vi "Teleop.vi"(10 "Match Info":T1={"Autonomous Elapsed Seconds"=0.0, "TeleOp Elapsed Seconds"=0.0, "Disabled Elapsed Seconds"=0.0, "Visited Autonomous"=FALSE, "Visited TeleOp"=FALSE, "Visited Disabled"=FALSE, "Autonomous Settings"={"Autonomous Style"=enum."Independent", "VI Refnum"=refnum}}, 11 "Call Context":T2) -> ()   [LabVIEW 2016]
doc: "This VI is called for each enabled TeleOp packet received from the DS. It is typically used to read from joysticks and other inputs and update I/O or setpoints for timed control loops. It should complete and return within 20 milliseconds or risk missing DS packets."
uses:
  <vilib>/Rock Robotics/WPI/DriverStation/WPI_DriverStationDerivedRobotMode.ctl
  <vilib>/Rock Robotics/WPI/DriverStation/WPI_DriverStationMatch Info.ctl
  <vilib>/Rock Robotics/WPI/ThirdParty/CanMotor/TalonSRX/WPI_CANTalonSRX_APIControlMode.ctl
  <vilib>/Rock Robotics/WPI/Utilities/WPI_GetSetVariantRefNum.vi
  <vilib>/Rock Robotics/Network Tables/NT Write Boolean Array.vi
  <vilib>/Rock Robotics/Network Tables/NT Write Numeric Array.vi
  <vilib>/Rock Robotics/Network Tables/NT Write String Array.vi
  <vilib>/Rock Robotics/Network Tables/NT Write Number.vi
  <vilib>/Rock Robotics/Network Tables/NT Read Number.vi
  Framework/Robot Global Data.vi
  <vilib>/Rock Robotics/Network Tables/NT Write Boolean.vi
panel:
  out "Percent Vbus?":bool
  out "Right Bumper Latched Driver":bool
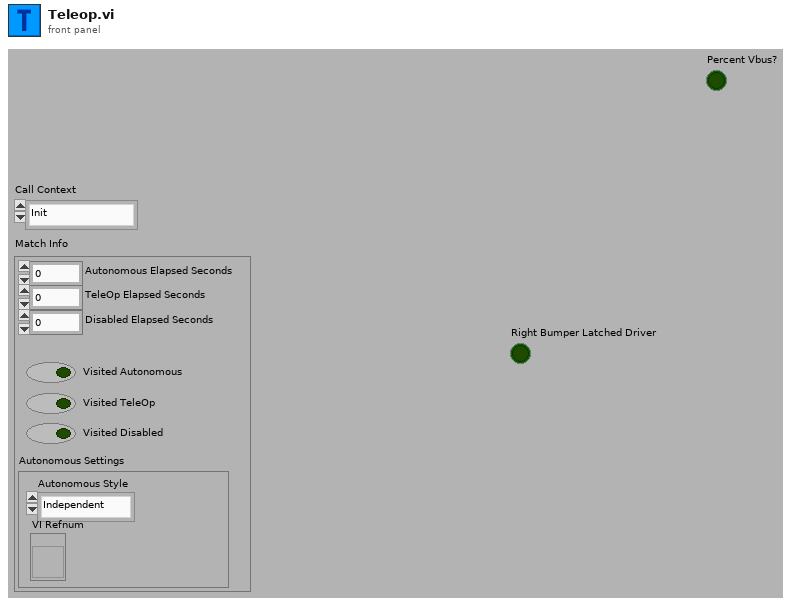
[diagram p1: front panel]
types:
  T1 = typedef "WPI_DriverStationMatch Info.ctl" = cluster{"Autonomous Elapsed Seconds":dbl, "TeleOp Elapsed Seconds":dbl, "Disabled Elapsed Seconds":dbl, "Visited Autonomous":bool, "Visited TeleOp":bool, "Visited Disabled":bool, "Autonomous Settings":cluster{"Autonomous Style":enum16{"Iterative", "Independent"}, "VI Refnum":refnum<vi>}}
  T2 = typedef "WPI_DriverStationDerivedRobotMode.ctl" = enum16{"Init", "Execute", "Stop"}
  T3 = typedef "WPI_JoystickDevRef.ctl" = cluster{"Device":T4}
  T4 = typedef "WPI_JoystickDeviceEnum.ctl" = enum16{"USB 0", "USB 1", "USB 2", "USB 3", "USB 4", "USB 5"}
  T5 = typedef "WPI_MotorControlDeviceRef.ctl" = cluster{"DeviceStatus":errorcluster, "Type":T6, "PWM":cluster{"PWM Channel":T7, "DeadBand":T8}, "CAN":cluster{"Device Number":u8, "SetOutput VI Ref":variant, "GetOutput VI Ref":variant, "Enable VI Ref":variant, "Disable VI Ref":variant, "Data":variant}, "Invert":bool}
  T6 = typedef "WPI_MotorControlType.ctl" = enum16{"PWM", "CAN"}
  T7 = typedef "FPGA_DIOPWMChannel.ctl" = enum8{"PWM 0", "PWM 1", "PWM 2", "PWM 3", "PWM 4", "PWM 5", "PWM 6", "PWM 7", "PWM 8", "PWM 9", "PWM MXP 0", "PWM MXP 1", "PWM MXP 2", "PWM MXP 3", "PWM MXP 4", "PWM MXP 5", "PWM MXP 6", "PWM MXP 7", "PWM MXP 8", "PWM MXP 9", "Invalid"}
  T8 = typedef "WPI_PWMDeadband.ctl" = cluster{"Name":string, "maxPositivePwm":i32, "minPositivePwm":i32, "centerPwm":i32, "maxNegativePwm":i32, "minNegativePwm":i32, "angularRange":u16}
  T9 = typedef "WPI_DigitalInputDevRef.ctl" = cluster{"DevStatus":errorcluster, "DIO Channel":T10}
  T10 = typedef "FPGA_DIOChannel.ctl" = enum8{"DIO 0", "DIO 1", "DIO 2", "DIO 3", "DIO 4", "DIO 5", "DIO 6", "DIO 7", "DIO 8", "DIO 9", "DIO MXP 0", "DIO MXP 1", "DIO MXP 2", "DIO MXP 3", "DIO MXP 4", "DIO MXP 5", "DIO MXP 6", "DIO MXP 7", "DIO MXP 8", "DIO MXP 9", "DIO MXP 10", "DIO MXP 11", "DIO MXP 12", "DIO MXP 13", "DIO MXP 14", "DIO MXP 15", "SPI Port CS1", "SPI Port CS2", "SPI Port CS3", "SPI Port MISO", "SPI Port MOSI", "Invalid"}
  T11 = typedef "WPI_RobotDriveDevRef.ctl" = cluster{"DevStatus":errorcluster, "Motors[]":T5[], "Square Inputs":bool, "Max Output":dbl}
  T12 = typedef "WPI_CANTalonSRX_APIControlMode.ctl" = enum8{"Percent VBus", "Speed", "Position", "Slave", "Unchanged / Invalid", "Voltage Compensation", "Current", "Motion Profile", "Motion Magic"}
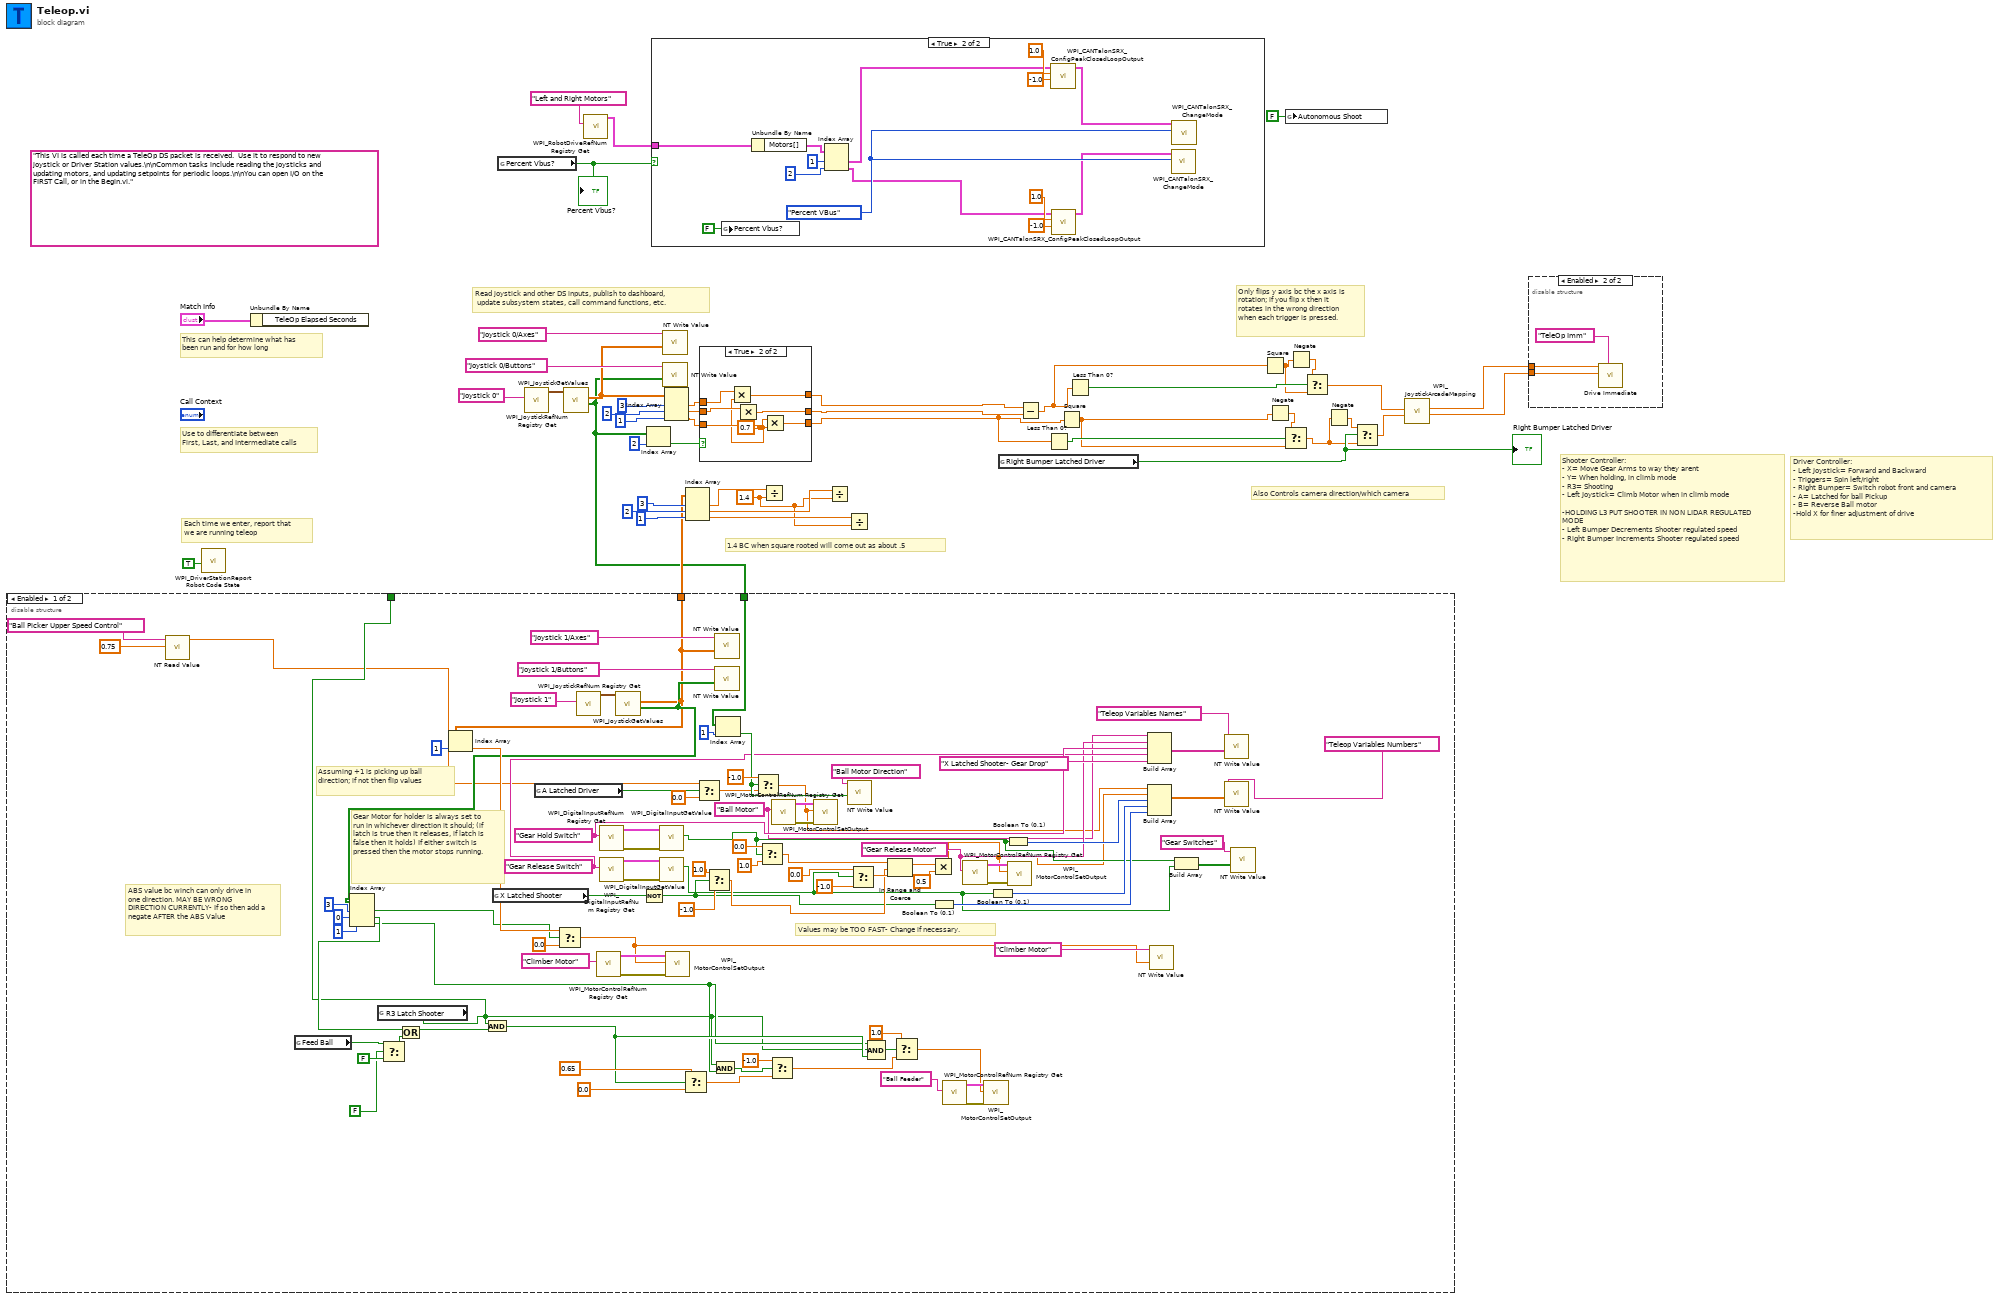
[diagram p0: block diagram]
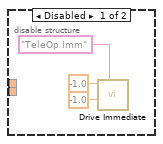
[diagram p4: hidden frame]
diagram:
  w13 = 1.4 ("y")
  (unwired) "This VI is called each time a TeleOp DS packet is received.  Use it to respond to new joystick or Driver Station values.\n\nCommon tasks include reading the joysticks and updating motors, and updating setpoints for periodic loops.\n\nYou can open I/O on the FIRST Call, or in the Begin.vi."
  # "1.4 BC when square rooted will come out as about .5"
  # "Driver Controller:\n- Left Joystick= Forward and Backward\n- Triggers= Spin left/right\n- Right Bumper= Switch robot front and camera\n- A= Latched for ball Pickup\n- B= Reverse Ball motor\n-Hold X for finer adjustment of drive"
  # "Shooter Controller:\n- X= Move Gear Arms to way they arent\n- Y= When holding, in climb mode\n- R3= Shooting\n- Left Joystick= Climb Motor when in climb mode\n\n-HOLDING L3 PUT SHOOTER IN NON LIDAR REGULATED MODE\n- Left Bumper Decrements Shooter regulated speed\n- Right Bumper Increments Shooter regulated speed"
  # "Only flips y axis bc the x axis is rotation; if you flip x then it rotates in the wrong direction when each trigger is pressed."
  # "Also Controls camera direction/which camera"
  # "Read joystick and other DS inputs, publish to dashboard,\n update subsystem states, call command functions, etc."
  # "Each time we enter, report that\nwe are running teleop"
  # "Use to differentiate between\nFirst, Last, and Intermediate calls"
  # "This can help determine what has\nbeen run and for how long"
  n1 = call <vilib>:"WPI_DriverStationReport Robot Code State.vi"("TeleOp"=TRUE ("Autonomous")) -> ()  [unwired: 10 in, 1 out]
  n2 = Unbundle By Name("Match Info") -> ()  [unwired: 1 out]
  n3 = global read "Robot Global Data.vi" "Percent Vbus?"() -> (w2:bool)
  "Percent Vbus?" <- w2
  n4 = call <vilib>:"WPI_JoystickRefNum Registry Get.vi"("refnum name"="Joystick 0") -> ("JoystickDevRef"=w42:T3)  [unwired: 1 in, 9 out]
  n5 = call <vilib>:"WPI_JoystickGetValues.vi"("JoystickDevRef"=w42) -> ("Buttons"=w12:bool[], "Axes"=w40:dbl[])  [unwired: 6 in, 3 out]
  n6 = disable-structure shown="Enabled" {
    disable-tunnel: w12 -> [w80 _]
    disable-tunnel: [w50 _] -> _
    disable-tunnel: [w66 _] -> w17
    frame Enabled {
      w110 = "Gear Release Switch" ("refnum name")
      w112 = "Gear Hold Switch" ("refnum name")
      w74 = "Gear Release Motor" ("refnum name")
      w73 = "Ball Motor" ("refnum name")
      # "ABS value bc winch can only drive in one direction. MAY BE WRONG DIRECTION CURRENTLY- If so then add a negate AFTER the ABS Value"
      # "Gear Motor for holder is always set to run in whichever direction it should; (if latch is true then it releases, if latch is false then it holds) If either switch is pressed then the motor stops running."
      # "Values may be TOO FAST- Change if necessary."
      # "Assuming +1 is picking up ball direction; if not then flip values"
      n7 = call-poly <vilib>:"NT Read Value.vi"("Default Value"=0.75, "Name"="Ball Picker Upper Speed Control") -> ("Numeric"=w49:dbl)  [unwired: 8 in, 1 out]
      n8 = global read "Robot Global Data.vi" "Feed Ball"() -> (w69:bool)
      n9 = global read "Robot Global Data.vi" "R3 Latch Shooter"() -> (w50:bool)
      n10 = Select(t=w69, s=FALSE ("AutoFeed Balls"), f=FALSE) -> (s? t:f=w70:bool)
      n11 = global read "Robot Global Data.vi" "X Latched Shooter"() -> (w81:bool)
      n12 = global read "Robot Global Data.vi" "A Latched Driver"() -> (w83:bool)
      n13 = call <vilib>:"WPI_JoystickRefNum Registry Get.vi"("refnum name"="Joystick 1") -> ("JoystickDevRef"=w133:T3)  [unwired: 1 in, 9 out]
      n14 = call <vilib>:"WPI_MotorControlRefNum Registry Get.vi"("refnum name"="Climber Motor") -> ("error out"=w120:errorcluster, "MotorControlDevRef"=w78:T5)  [unwired: 9 in]
      n15 = call <vilib>:"WPI_DigitalInputRefNum Registry Get.vi"("refnum name"=w112) -> ("error out"=w124:errorcluster, "DigitalInputDevRef"=w123:T9)  [unwired: 9 in]
      n16 = call <vilib>:"WPI_DigitalInputRefNum Registry Get.vi"("refnum name"=w110) -> ("error out"=w122:errorcluster, "DigitalInputDevRef"=w121:T9)  [unwired: 9 in]
      n17 = call <vilib>:"WPI_JoystickGetValues.vi"("JoystickDevRef"=w133) -> ("Buttons"=w86:bool[], "Axes"=w66:dbl[])  [unwired: 6 in, 3 out]
      n18 = Index Array(array=w86, index #1=3 ("index"), index #2=0 ("index"), index #3=1 ("index")) -> (element #1=w85:bool, element #2=w75:bool, element #3=w51:bool)
      n19 = Or(x=w75, y=w70) -> (x .or. y?=w71:bool)
      n20 = Index Array(array=w66, index=1) -> (element=w88:dbl)
      n21 = And(x=w50, y=w71) -> (x .and. y?=w53:bool)
      n22 = Select(t=w88, s=w85, f=0.0) -> (s? t:f=w77:dbl)
      n23 = Not(x=w81) -> (.not. x?=w79:bool)
      n24 = call <vilib>:"WPI_DigitalInputGetValue.vi"("error in (no error)"=w124, "DigitalInputDevRef"=w123) -> ("Value"=w93:bool)  [unwired: 7 in, 2 out]
      n25 = call <vilib>:"WPI_DigitalInputGetValue.vi"("error in (no error)"=w122, "DigitalInputDevRef"=w121) -> ("Value"=w92:bool)  [unwired: 7 in, 2 out]
      n26 = call <vilib>:"WPI_MotorControlSetOutput.vi"("error in (no error)"=w120, "Output"=w77, "MotorControlDevRef"=w78) -> ()  [unwired: 6 in, 3 out]
      n27 = Select(t=0.65 ("Ball Feeder Speed"), s=w53, f=0.0) -> (s? t:f=w60:dbl)
      n28 = Select(t=w49, s=w83, f=0.0) -> (s? t:f=w84:dbl)
      n29 = Select(t=1.0, s=w79, f=-1.0) -> (s? t:f=w94:dbl)
      n30 = And(x=w50, y=w51) -> (x .and. y?=w52:bool)
      n31 = call-poly <vilib>:"NT Write Value.vi"("Numeric Array"=w66, "Name"="Joystick 1/Axes") -> ()  [unwired: 9 in, 1 out]
      n32 = call-poly <vilib>:"NT Write Value.vi"("Boolean Array"=w86, "Name"="Joystick 1/Buttons") -> ()  [unwired: 9 in, 1 out]
      n33 = Index Array(array=w80, index=1) -> (element=w118:bool)
      n34 = Select(t=-1.0 ("Backward"), s=w118, f=w84) -> (s? t:f=w46:dbl)
      n35 = Select(t=0.0, s=w93, f=1.0) -> (s? t:f=w95:dbl)
      n36 = Select(t=-1.0, s=w52, f=w60) -> (s? t:f=w55:dbl)
      n37 = call <vilib>:"WPI_MotorControlRefNum Registry Get.vi"("refnum name"=w73) -> ("error out"=w130:errorcluster, "MotorControlDevRef"=w129:T5)  [unwired: 9 in]
      n38 = call <vilib>:"WPI_MotorControlSetOutput.vi"("error in (no error)"=w130, "Output"=w46, "MotorControlDevRef"=w129) -> ()  [unwired: 6 in, 3 out]
      n39 = call-poly <vilib>:"NT Write Value.vi"("Boolean"=w118, "Name"="Ball Motor Direction") -> ()  [unwired: 9 in, 1 out]
      n40 = Select(t=0.0, s=w92, f=-1.0) -> (s? t:f=w100:dbl)
      n41 = Compound Arithmetic op=AND(w51, w50, w53) -> (w56:bool)
      n42 = In Range and Coerce(upper limit=w95, x=w94, lower limit=w100) -> (coerced(x)=w91:dbl)  [unwired: 1 out]
      n43 = Select(t=1.0, s=w56, f=w55) -> (s? t:f=w57:dbl)
      n44 = Multiply(x=w91, y=0.5) -> (x*y=w72:dbl)
      n45 = Boolean To (0,1)(Boolean=w79) -> (0, 1=w107:i16)
      n46 = call <vilib>:"WPI_MotorControlRefNum Registry Get.vi"("refnum name"="Ball Feeder") -> ("error out"=w65:errorcluster, "MotorControlDevRef"=w64:T5)  [unwired: 9 in]
      n47 = call <vilib>:"WPI_MotorControlRefNum Registry Get.vi"("refnum name"=w74) -> ("error out"=w126:errorcluster, "MotorControlDevRef"=w125:T5)  [unwired: 9 in]
      n48 = call <vilib>:"WPI_MotorControlSetOutput.vi"("error in (no error)"=w65, "Output"=w57, "MotorControlDevRef"=w64) -> ()  [unwired: 6 in, 3 out]
      n49 = Boolean To (0,1)(Boolean=w92) -> (0, 1=w109:i16)
      n50 = Boolean To (0,1)(Boolean=w93) -> (0, 1=w111:i16)
      n51 = call <vilib>:"WPI_MotorControlSetOutput.vi"("error in (no error)"=w126, "Output"=w72, "MotorControlDevRef"=w125) -> ()  [unwired: 6 in, 3 out]
      n52 = Build Array(w73, w74, w112, w110, "X Latched Shooter- Gear Drop") -> (w115:string[])
      n53 = Build Array(w46, w72, w111, w109, w107) -> (w114:dbl[])
      n54 = call-poly <vilib>:"NT Write Value.vi"("Numeric"=w77, "Name"="Climber Motor") -> ()  [unwired: 9 in, 1 out]
      n55 = Build Array(w93, w92) -> (w104:bool[])
      n56 = call-poly <vilib>:"NT Write Value.vi"("String Array"=w115, "Name"="Teleop Variables Names") -> ()  [unwired: 9 in, 1 out]
      n57 = call-poly <vilib>:"NT Write Value.vi"("Numeric Array"=w114, "Name"="Teleop Variables Numbers") -> ()  [unwired: 9 in, 1 out]
      n58 = call-poly <vilib>:"NT Write Value.vi"("Boolean Array"=w104, "Name"="Gear Switches") -> ()  [unwired: 9 in, 1 out]
    }
    frame Disabled {
    }
  }
  n59 = call <vilib>:"WPI_RobotDriveRefNum Registry Get.vi"("refnum name"="Left and Right Motors") -> ("RobotDriveDevRef"=w5:T11)  [unwired: 9 in, 1 out]
  n60 = Index Array(array=w12, index=2) -> (element=w7:bool)
  n61 = case shown="True" w2 {
    tunnel: w5 -> [_ w143]
    frame False {
    }
    frame True {
      w145 = WPI_CANTalonSRX_APIControlMode."Percent VBus" ("Control Mode")
      n62 = global write "Robot Global Data.vi" "Percent Vbus?"(FALSE ("Percent Vbus?")) -> ()
      n63 = Unbundle By Name(w143) -> ("Motors[]"=w148:T5[])
      n64 = Index Array(array=w148, index #1=1 ("index"), index #2=2 ("index")) -> (element #1=w137:T5, element #2=w136:T5)
      n65 = call <vilib>:"WPI_CANTalonSRX_ConfigPeakClosedLoopOutput.vi"("Reverse Peak Output"=-1.0, "Forward Peak Output"=1.0, "CAN Talon SRX Ref"=w137) -> ("CAN Talon SRX Ref"=w138:T5)  [unwired: 7 in, 1 out]
      n66 = call <vilib>:"WPI_CANTalonSRX_ConfigPeakClosedLoopOutput.vi"("Reverse Peak Output"=-1.0, "Forward Peak Output"=1.0, "CAN Talon SRX Ref"=w136) -> ("CAN Talon SRX Ref"=w135:T5)  [unwired: 7 in, 1 out]
      n67 = call <vilib>:"WPI_CANTalonSRX_ChangeMode.vi"("Control Mode"=w145, "CAN Talon SRX Ref"=w135) -> ()  [unwired: 8 in, 2 out]
      n68 = call <vilib>:"WPI_CANTalonSRX_ChangeMode.vi"("Control Mode"=w145, "CAN Talon SRX Ref"=w138) -> ()  [unwired: 8 in, 2 out]
    }
  }
  n69 = call-poly <vilib>:"NT Write Value.vi"("Numeric Array"=w40, "Name"="Joystick 0/Axes") -> ()  [unwired: 9 in, 1 out]
  n70 = call-poly <vilib>:"NT Write Value.vi"("Boolean Array"=w12, "Name"="Joystick 0/Buttons") -> ()  [unwired: 9 in, 1 out]
  n71 = Index Array(array=w40, index #1=3 ("index"), index #2=2 ("index"), index #3=1 ("index")) -> (element #1=w10:dbl, element #2=w9:dbl, element #3=w8:dbl)
  n72 = Index Array(array=w17, index #1=3 ("index"), index #2=2 ("index"), index #3=1 ("index")) -> (element #1=w14:dbl, element #2=w15:dbl, element #3=w16:dbl)
  n73 = case shown="True" w7 {
    tunnel: w10 -> [w151 w158]
    tunnel: w9 -> [w150 w157]
    tunnel: w8 -> [w149 w156]
    tunnel: [w151 w154] -> w23
    tunnel: [w150 w153] -> w22
    tunnel: [w149 w152] -> w21
    frame False {
    }
    frame True {
      w155 = 0.7 ("y")
      n74 = Multiply(x=w158, y=w155) -> (x*y=w154:dbl)
      n75 = Multiply(x=w157, y=w155) -> (x*y=w153:dbl)
      n76 = Multiply(x=w156, y=w155) -> (x*y=w152:dbl)
    }
  }
  n77 = Divide(x=w14, y=w13) -> ()  [unwired: 1 out]
  n78 = Divide(x=w15, y=w13) -> ()  [unwired: 1 out]
  n79 = Divide(x=w16, y=w13) -> ()  [unwired: 1 out]
  n80 = global read "Robot Global Data.vi" "Right Bumper Latched Driver"() -> (w33:bool)
  "Right Bumper Latched Driver" <- w33
  n81 = Subtract(x=w23, y=w22) -> (x-y=w29:dbl)
  n82 = Less Than 0?(x=w21) -> (x < 0?=w27:bool)
  n83 = Square(x=w21) -> (x^2=w25:dbl)
  n84 = Less Than 0?(x=w29) -> (x < 0?=w32:bool)
  n85 = Square(x=w29) -> (x^2=w30:dbl)
  n86 = Negate(x=w25) -> (-x=w26:dbl)
  n87 = Select(t=w26, s=w27, f=w25) -> (s? t:f=w24:dbl)
  n88 = global write "Robot Global Data.vi" "Autonomous Shoot"(FALSE ("Autonomous Shoot")) -> ()
  n89 = Negate(x=w30) -> (-x=w31:dbl)
  n90 = Select(t=w31, s=w32, f=w30) -> (s? t:f=w28:dbl)
  n91 = Negate(x=w24) -> (-x=w38:dbl)
  n92 = Select(t=w38, s=w33, f=w24) -> (s? t:f=w37:dbl)
  n93 = call <vilib>:"WPI_JoystickArcadeMapping.vi"("Y axis value"=w37, "X axis value"=w28) -> ("Right Motor Value"=w3:dbl, "Left Motor Value"=w4:dbl)  [unwired: 8 in]
  n94 = disable-structure shown="Enabled" {
    disable-tunnel: w4 -> [_ w163]
    disable-tunnel: w3 -> [_ w162]
    frame Disabled {
      n95 = call "Drive Immediate.vi"("Description"="TeleOp Imm", "Right Setpoint"=-1.0, "Left Setpoint"=-1.0) -> ()  [unwired: 8 in, 1 out]
    }
    frame Enabled {
      n96 = call "Drive Immediate.vi"("Description"="TeleOp Imm", "Right Setpoint"=w162, "Left Setpoint"=w163) -> ()  [unwired: 8 in, 1 out]
    }
  }
